vi "Event Handle Loop_Initialize.vi"(8 "error in (no error)":errorcluster, 11 "QTab Class in":refnum<class "QTab Class.lvclass">) -> (0 "error out":errorcluster, 2 "Event Refnum":refnum<event-registration>, 3 "QTab Class out":refnum<class "QTab Class.lvclass">)   [LabVIEW 2020, in "QTab.lvlib" / "QTab Class.lvclass"]
uses:
  QTab Class.lvclass
  QMenu Class/Notifier User Event.ctl
  QMenu Class/Active Event Data.ctl
  QMenu Class/Close Event Data.ctl
  QMenu Class/Drag Event Data.ctl
  Command Data.ctl
  Command.ctl
  QTab Class.lvclass/QTab Class.ctl
  QMenu Class/QMenu Class.lvclass/QMenu Class.ctl
  QMenu Class/Read Notifier User Event.vi
  QMenu Class/Write Close Timeout.vi
  QMenu Class/Write Drag Timeout.vi
  QMenu Class/QMenu Class.lvclass
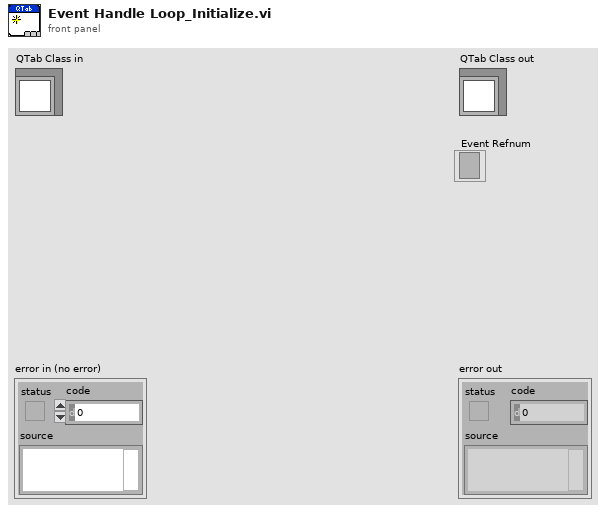
[diagram p1: front panel]
types:
  T1 = typedef "QTab.lvlib/QTab Class.lvclass/Command.ctl" = enum16{"Startup", "Add Page", "Close All Page", "Set Page Attribute", "Pop-out", "Merage", "Insert", "Stop"}
  T2 = typedef "QTab.lvlib/QMenu Class.lvclass/Notifier User Event.ctl" = cluster{"Active User Event":refnum<user-event>, "Close User Event":refnum<user-event>, "Drag User Event":refnum<user-event>}
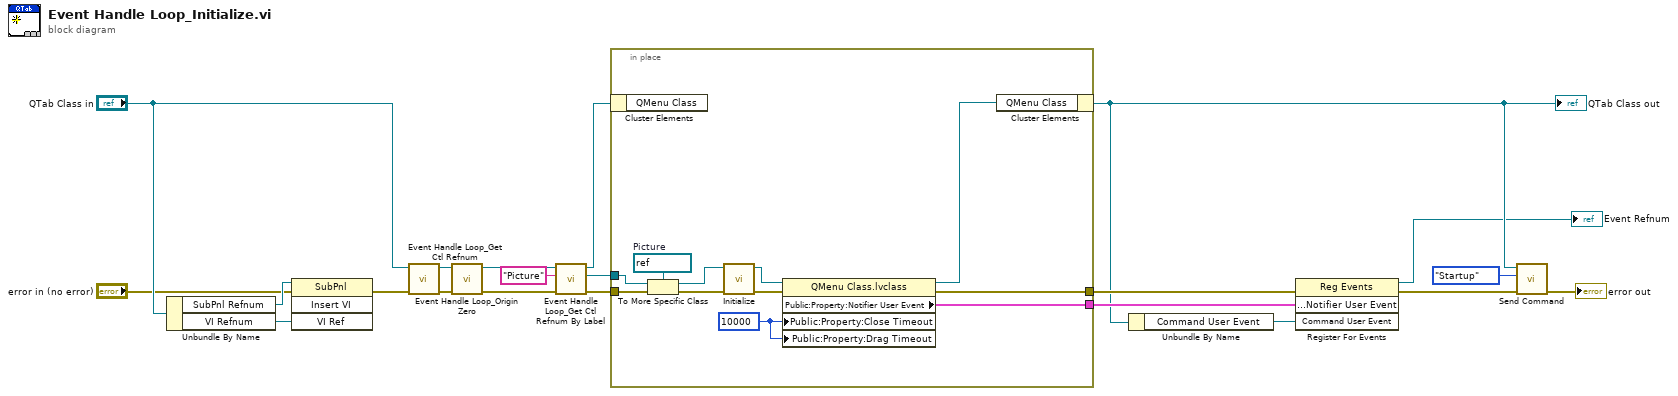
[diagram p0: block diagram]
diagram:
  n1 = Unbundle By Name("QTab Class in") -> ("SubPnl Refnum"=w14:refnum<vi>, "VI Refnum"=w15:refnum<vi>)
  n2 = invoke class="SubPnl" method="Insert VI"(reference=w14, error in="error in (no error)", "VI Ref"=w15) -> (error out=w12:errorcluster)  [unwired: 1 in, 3 out]
  n3 = call "Event Handle Loop_Get Ctl Refnum.vi"("error in (no error)"=w12, "QTab Class in"="QTab Class in") -> ("error out"=w21:errorcluster, "QTab Class out"=w20:refnum<class "QTab Class.lvclass">)  [unwired: 8 in]
  n4 = call "Event Handle Loop_Origin Zero.vi"("error in (no error)"=w21, "QTab Class in"=w20) -> ("error out"=w5:errorcluster, "QTab Class out"=w6:refnum<class "QTab Class.lvclass">)  [unwired: 8 in]
  n5 = call "Event Handle Loop_Get Ctl Refnum By Label.vi"("error in (no error)"=w5, "Label"="Picture", "QTab Class in"=w6) -> ("error out"=w17:errorcluster, "Ctl Refnum"=w16:refnum<vi>, "QTab Class out"=w18:refnum<class "QTab Class.lvclass">)  [unwired: 6 in]
  n6 = in-place {
    in-place-border: w17 -> [w29]
    in-place-border: w16 -> [w28]
    in-place-border: [w24] -> w10
    in-place-border: [w23] -> w9
    w22 = 10000 ("Close Timeout")
    w30 = refnum<vi> refnum  # Picture
    n7 = in-place-cluster #1(w18) -> ()  [unwired: 1 out]
    n8 = To More Specific Class(target class=w30, reference=w28, error in=w29) -> (specific class reference=w32:refnum<vi>, error out=w31:errorcluster)
    n9 = call "Initialize.vi"("error in (no error)"=w31, "Pict Refnum"=w32) -> ("error out"=w27:errorcluster, "QMenu Class out"=w26:refnum<class "QMenu Class.lvclass">)  [unwired: 8 in]
    n10 = property class="QMenu Class.lvclass"(reference=w26, error in=w27, "Public:Property:Close Timeout"=w22, "Public:Property:Drag Timeout"=w22) -> (reference out=w25:refnum<class "QMenu Class.lvclass">, error out=w24:errorcluster, "Public:Property:Notifier User Event"=w23:T2)
    n11 = in-place-cluster #1("QMenu Class"=w25) -> (w3:refnum<class "QTab Class.lvclass">)
  }
  "QTab Class out" <- w3
  n12 = Unbundle By Name(w3) -> ("Command User Event"=w8:refnum<user-event>)
  n13 = register-events(error in=w10, w9, w8) -> (reference out=→"Event Refnum":refnum<event-registration>, error out=w4:errorcluster)  [unwired: 1 in]
  n14 = call "Send Command.vi"("error in (no error)"=w4, "Command"=Command."Startup", "QTab Class in"=w3) -> ("error out"=→"error out":errorcluster)  [unwired: 7 in, 1 out]
